vi "HierarchyString.vi"(8 "Error":errorcluster, 11 "ProjectItem":refnum<vi>) -> (0 "Error":errorcluster, 3 "Project Path":string)   [LabVIEW 2021, in "Tree.lvlib" / "Tree.lvclass"]
uses:
  Tree.lvclass
panel:
  # "Формирует строку иерархии расположения\nискомого объекта в проекте.\nПервый элемент - высший\nПоследний элемент - низший"
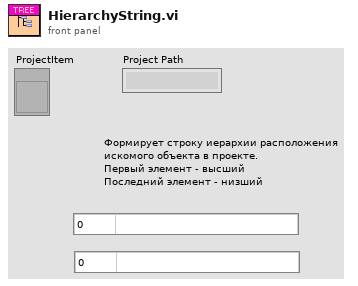
[diagram p1: front panel]
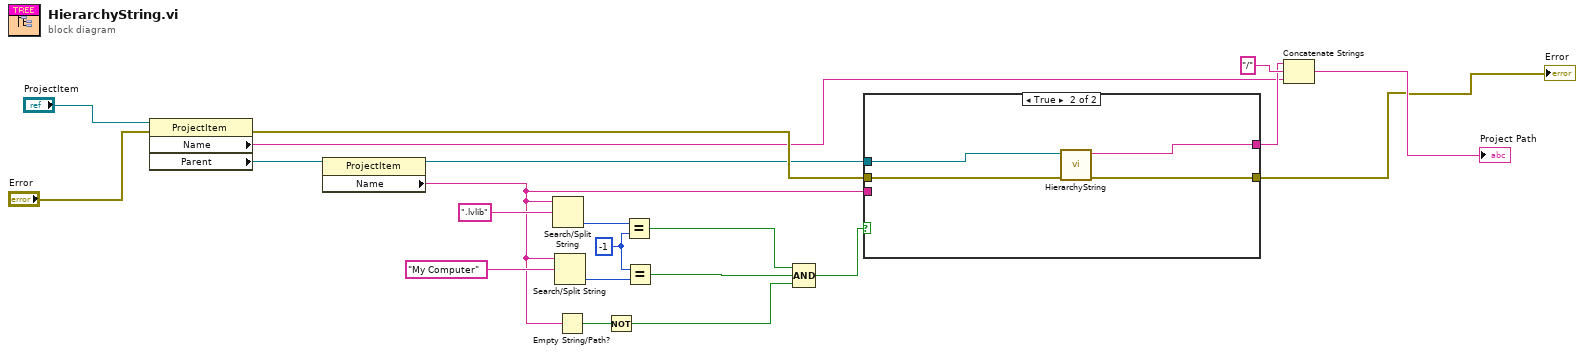
[diagram p0: block diagram]
diagram:
  w12 = -1 ("y")
  n1 = property class="ProjectItem"(reference="ProjectItem", error in="Error") -> (error out=w19:errorcluster, "Name"=w4:string, "Parent"=w3:refnum<vi>)  [unwired: 1 out]
  n2 = property class="ProjectItem"(reference=w3) -> (reference out=w2:refnum<vi>, "Name"=w1:string)  [unwired: 1 in, 1 out]
  n3 = Search/Split String(string=w1, search string/char (-)=".lvlib") -> (offset of match=w14:i32)  [unwired: 1 in, 2 out]
  n4 = Search/Split String(string=w1, search string/char (-)="My Computer") -> (offset of match=w13:i32)  [unwired: 1 in, 2 out]
  n5 = Empty String/Path?(string/path=w1) -> (empty?=w11:bool)
  n6 = Not(x=w11) -> (.not. x?=w7:bool)
  n7 = Equal?(x=w14, y=w12) -> (x = y?=w10:bool)
  n8 = Equal?(x=w12, y=w13) -> (x = y?=w9:bool)
  n9 = Compound Arithmetic op=AND(w10, w9, w7) -> (w8:bool)
  n10 = case shown="True" w8 {
    tunnel: w2 -> [_ w27]
    tunnel: [w22 w26] -> w5
    tunnel: w19 -> [w23 w25]
    tunnel: [w23 w24] -> w17
    tunnel: w1 -> [w22 _]
    frame False {
    }
    frame True {
      n11 = call "HierarchyString.vi"("Error"=w25, "ProjectItem"=w27) -> ("Error"=w24:errorcluster, "Project Path"=w26:string)  [unwired: 8 in]
    }
  }
  "Error" <- w17
  n12 = Concatenate Strings(w5, "/" ("string"), w4) -> (→"Project Path":string)
